vi "test_array_blocks.vi"() -> ()   [LabVIEW 2009]
panel:
  out "x = y?":bool
  out "element":u8
  out "output array":u8[](array[numeric])
  in  "new element/subarray":u8
  in  "column":u8
  in  "row":u8
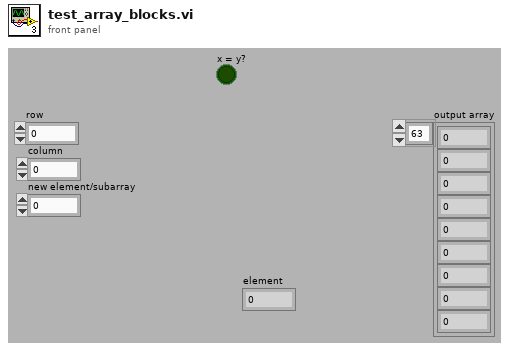
[diagram p1: front panel]
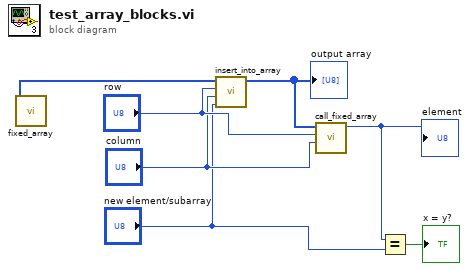
[diagram p0: block diagram]
diagram:
  n1 = call "fixed_array.vi"() -> ("Array"=w7:u8[])  [unwired: 11 in]
  n2 = call "insert_into_array.vi"("new element/subarray"="new element/subarray", "column"="column", "row"="row", "array"=w7) -> ("output array"=w6:u8[])  [unwired: 7 in]
  "output array" <- w6
  n3 = call "call_fixed_array.vi"("column"="column", "row"="row", "array"=w6) -> ("element"=w3:u8)  [unwired: 8 in]
  "element" <- w3
  n4 = Equal?(x=w3, y="new element/subarray") -> (x = y?=→"x = y?":bool)
